vi "Drop Message Core.vi"(11 "Reply Msg Generic Image in":refnum<class "Reply Msg Generic Image Arr.lvclass">) -> ()   [LabVIEW 2025, in "Reply Msg Generic Image Arr.lvclass"]
doc: "Children of Message should override this method if they have behavior when the Actor receiving this message stops running before the message gets handled. Predominantly, this is overridden by Reply Message.lvclass in order to tell the waiting caller that there will never be a reply from the callee. This method probably does not need to be overridden by any other class."
uses:
  Reply Msg Generic Image Arr.lvclass
  Reply Msg Generic Image Arr.lvclass/Reply Msg Generic Image Arr.ctl
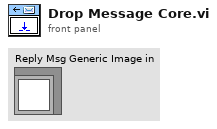
[diagram p1: front panel]
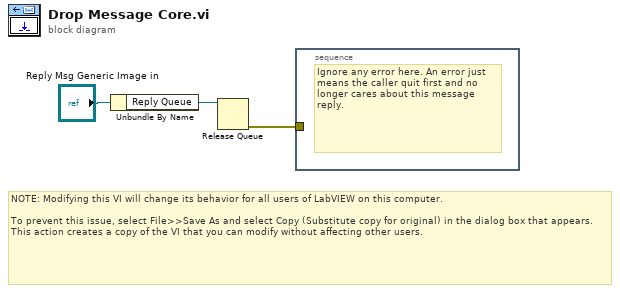
[diagram p0: block diagram]
diagram:
  # "NOTE: Modifying this VI will change its behavior for all users of LabVIEW on this computer.\n\nTo prevent this issue, select File>>Save As and select Copy (Substitute copy for original) in the dialog box that appears. This action creates a copy of the VI that you can modify without affecting other users."
  n1 = Unbundle By Name("Reply Msg Generic Image in") -> ("Reply Queue"=w2:refnum<queue>)
  n2 = Release Queue(queue=w2) -> (error out=w1:errorcluster)  [unwired: 2 in, 2 out]
  n3 = stacked-sequence {
    tunnel: w1 -> [_]
    frame #0 {
      # "Ignore any error here. An error just means the caller quit first and no longer cares about this message reply."
    }
  }
